vi "Stop Core.vi"(10 "final error code":i32, 11 "Common Measurements Interface in":refnum<class "Common Measurements Interface.lvclass">) -> (3 "Common Measurements Interface out":refnum<class "Common Measurements Interface.lvclass">)   [LabVIEW 2015, in "Common Measurements Interface.lvclass"]
uses:
  Common Measurements Interface.lvclass
  <vilib>/ActorFramework/Actor/Actor.lvclass/Actor.ctl
  Common Measurements Interface.lvclass/Common Measurements Interface.ctl
  <vilib>/ActorFramework/Message Enqueuer/Message Enqueuer.lvclass/Message Enqueuer.ctl
  <vilib>/ActorFramework/Message Enqueuer/Enqueue.vi
  <vilib>/ActorFramework/Message Priority Queue/Priority Enqueue.vi
  Mag Lab Measure Interface/Interface with menu/Interface with menu.lvclass
  <vilib>/ActorFramework/Stop Msg/Stop Msg.lvclass
  <vilib>/ActorFramework/Actor/Actor.lvclass
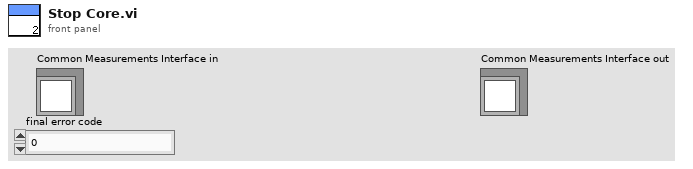
[diagram p1: front panel]
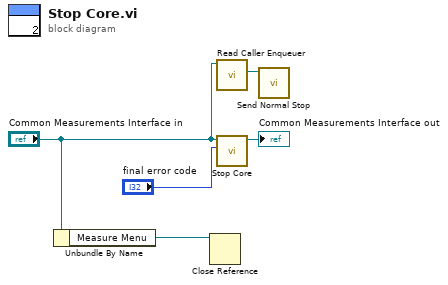
[diagram p0: block diagram]
diagram:
  n1 = Unbundle By Name("Common Measurements Interface in") -> ("Measure Menu"=w1:refnum<vi>)
  n2 = Close Reference(reference=w1) -> ()  [unwired: 1 in, 1 out]
  n3 = call <vilib>:"Read Caller Enqueuer.vi"("Actor"="Common Measurements Interface in") -> ("Caller Enqueuer"=w3:refnum<class "Message Enqueuer.lvclass">)  [unwired: 10 in]
  n4 = call-parent "Stop Core.vi"("final error code"="final error code", "Interface with menu in"="Common Measurements Interface in") -> ("Interface with menu out"=→"Common Measurements Interface out":refnum<class "Common Measurements Interface.lvclass">)  [unwired: 9 in]
  n5 = call <vilib>:"Send Normal Stop.vi"("Message Enqueuer"=w3) -> ()  [unwired: 10 in, 1 out]
